vi "dStr neuron.vi"(1 "In 4":bool, 2 "In 3":bool, 3 "In 2":bool, 4 "In":bool) -> (0 "Out":bool)   [LabVIEW 2014]
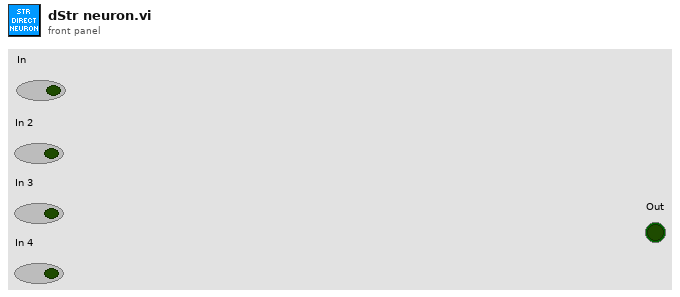
[diagram p1: front panel]
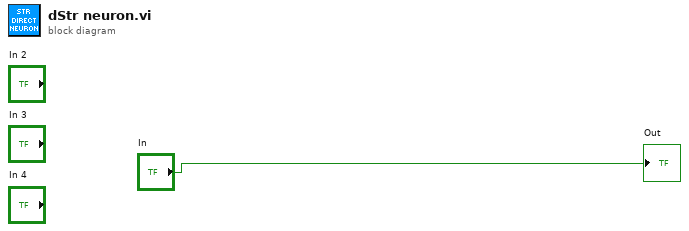
[diagram p0: block diagram]
diagram:
  "Out" <- "In"
